vi "test SSL Client Valid Socket FD.vi"(8 "error in (no error)":errorcluster, 11 "TestCase in":refnum<class "test SSL Client.lvclass">) -> (0 "error out":errorcluster, 3 "TestCase out":refnum<class "test SSL Client.lvclass">)   [LabVIEW 2013, in "test SSL Client.lvclass"]
uses:
  test SSL Client.lvclass
  <vilib>/addons/_JKI Toolkits/VI Tester/TestCase.llb/TestCase.lvclass
  SSL_Lib/BIO/BIO.lvclass
  SSL_Lib/SSL-Context/SSL-Context.lvclass
  SSL_Lib/SSL/SSL.lvclass
  SSL_Lib/SSL/SSL_Mode.ctl
  suite SSL Client/suite SSL Client/SSL Context.vi
  suite SSL Client/suite SSL Client/suite SSL Client.lvclass
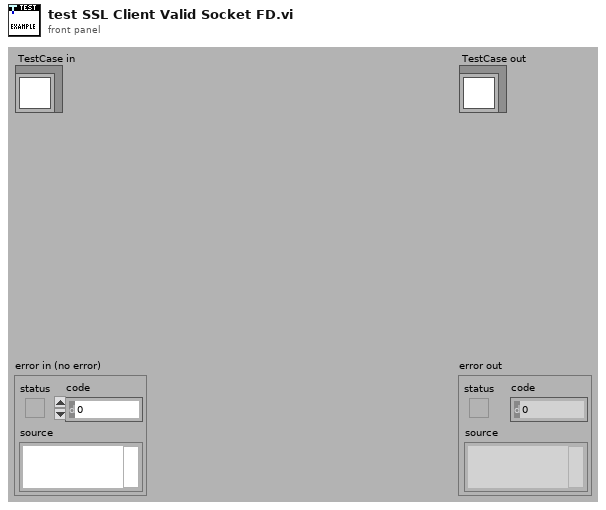
[diagram p1: front panel]
types:
  T1 = typedef "SSL_Lib.lvlib/SSL.lvclass/SSL_Mode.ctl" = i32
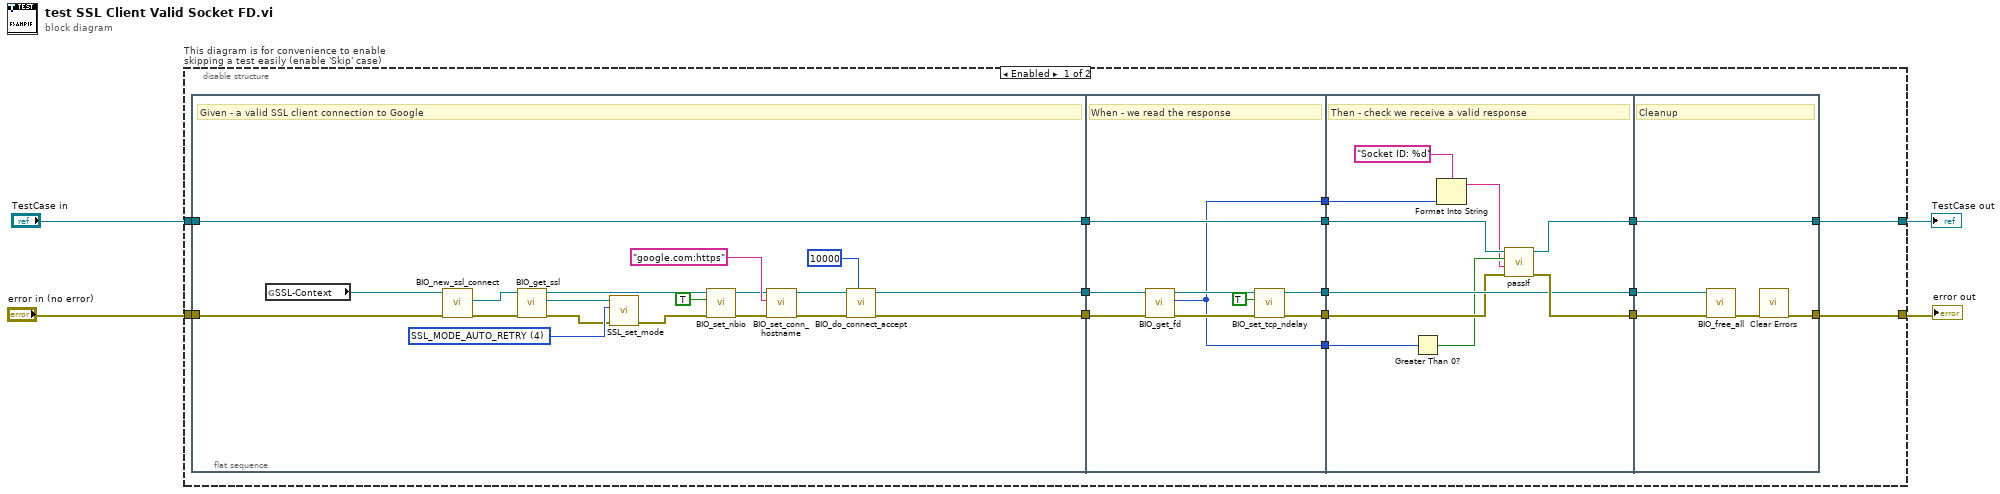
[diagram p0: block diagram]
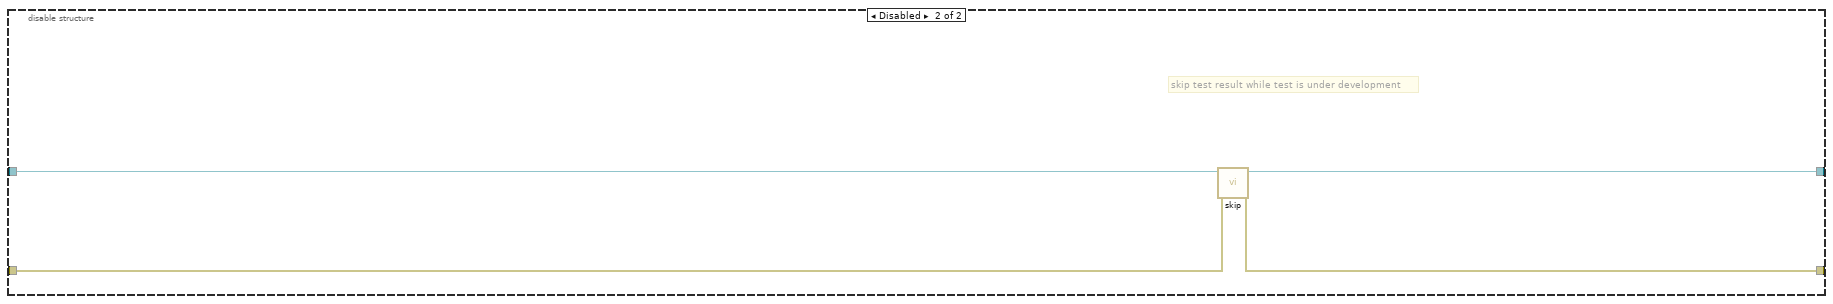
[diagram p2: hidden frame]
diagram:
  n1 = disable-structure "This diagram is for convenience to enable skipping a test easily (enable 'Skip' case)" shown="Enabled" {
    disable-tunnel: "TestCase in" -> [w14 w66]
    disable-tunnel: [w13 w64] -> w1
    disable-tunnel: [w12 w65] -> w3
    disable-tunnel: "error in (no error)" -> [w15 w63]
    frame Enabled {
      n2 = flat-sequence {
        tunnel: w15 -> [w28]
        tunnel: w14 -> [w35]
        tunnel: [w35] -> w19
        tunnel: [w21] -> w9
        tunnel: [w20] -> w8
        tunnel: [w47] -> w18
        tunnel: w19 -> [w47]
        tunnel: [w46] -> w11
        tunnel: w9 -> [w45]
        tunnel: w8 -> [w42]
        tunnel: [w41] -> w7
        tunnel: [w41] -> w6
        tunnel: [w39] -> w5
        tunnel: [w56] -> w17
        tunnel: [w55] -> w16
        tunnel: w18 -> [w57]
        tunnel: w11 -> [w54]
        tunnel: [w54] -> w10
        tunnel: w7 -> [w53]
        tunnel: w6 -> [w52]
        tunnel: w5 -> [w51]
        tunnel: [w58] -> w12
        tunnel: [w62] -> w13
        tunnel: w17 -> [w62]
        tunnel: w16 -> [w61]
        tunnel: w10 -> [w59]
        frame #0 {
          w30 = T1 4 items=["None"=0, "SSL_MODE_ENABLE_PARTIAL_WRITE"=1, "SSL_MODE_ACCEPT_MOVING_WRITE_BUFFER"=2, "SSL_MODE_AUTO_RETRY"=4, "SSL_MODE_RELEASE_BUFFERS"=16, "SSL_MODE_SEND_FALLBACK_SCSV"=128] ("Mode")
          # "Given - a valid SSL client connection to Google"
          n3 = global read "SSL Context.vi" "SSL-Context"() -> (w27:refnum<class "SSL-Context.lvclass">)
          n4 = call "BIO_new_ssl_connect.vi"("error in (no error)"=w28, "SSL-Context in"=w27) -> ("error out"=w32:errorcluster, "BIO out"=w33:refnum<class "BIO.lvclass">)  [unwired: 7 in, 1 out]
          n5 = call "BIO_get_ssl.vi"("error in (no error)"=w32, "BIO in"=w33) -> ("error out"=w29:errorcluster, "SSL out"=w31:refnum<class "SSL.lvclass">, "BIO out"=w22:refnum<class "BIO.lvclass">)  [unwired: 7 in]
          n6 = call "SSL_set_mode.vi"("error in (no error)"=w29, "Mode"=w30, "SSL in"=w31) -> ("error out"=w25:errorcluster)  [unwired: 7 in, 1 out]
          n7 = call "BIO_set_nbio.vi"("error in (no error)"=w25, "Non-Blocking?"=TRUE, "BIO in"=w22) -> ("error out"=w23:errorcluster, "BIO out"=w24:refnum<class "BIO.lvclass">)  [unwired: 7 in]
          n8 = call "BIO_set_conn_hostname.vi"("error in (no error)"=w23, "Hostname"="google.com:https", "BIO in"=w24) -> ("error out"=w37:errorcluster, "BIO out"=w34:refnum<class "BIO.lvclass">)  [unwired: 7 in]
          n9 = call "BIO_do_connect_accept.vi"("Timeout (10000ms)"=u32 10000, "error in (no error)"=w37, "BIO in"=w34) -> ("error out"=w21:errorcluster, "BIO out"=w20:refnum<class "BIO.lvclass">)  [unwired: 7 in]
        }
        frame #1 {
          # "When - we read the response"
          n10 = call "BIO_get_fd.vi"("error in (no error)"=w45, "BIO in"=w42) -> ("error out"=w44:errorcluster, "socket fd"=w41:i32, "BIO out"=w43:refnum<class "BIO.lvclass">)  [unwired: 7 in]
          n11 = call "BIO_set_tcp_ndelay.vi"("error in (no error)"=w44, "No Delay?"=TRUE, "BIO in"=w43) -> ("error out"=w39:errorcluster, "BIO out"=w46:refnum<class "BIO.lvclass">)  [unwired: 7 in]
        }
        frame #2 {
          # "Then - check we receive a valid response"
          n12 = Greater Than 0?(x=w52) -> (x > 0?=w50:bool)
          n13 = Format Into String(format string="Socket ID: %d", w53) -> (resulting string=w48:string)  [unwired: 2 in, 1 out]
          n14 = call-dynamic "passIf.vi"("error in (no error)"=w51, "message (\"\")"=w48, "pass"=w50, "TestCase in"=w57) -> ("error out"=w55:errorcluster, "TestCase out"=w56:refnum<class "test SSL Client.lvclass">)  [unwired: 6 in]
        }
        frame #3 {
          # "Cleanup"
          n15 = call "BIO_free_all.vi"("error in (no error)"=w61, "BIO in"=w59) -> ("error out"=w60:errorcluster)  [unwired: 9 in]
          n16 = call <vilib>:"Clear Errors.vi"("error in (no error)"=w60) -> ("error out"=w58:errorcluster)  [unwired: 5 in, 1 out]
        }
      }
    }
    frame Disabled {
      # "skip test result while test is under development"
      n17 = call <vilib>:"skip.vi"("error in (no error)"=w63, "TestCase in"=w66) -> ("error out"=w65:errorcluster, "TestCase out"=w64:refnum<class "test SSL Client.lvclass">)  [unwired: 8 in]
    }
  }
  "error out" <- w3
  "TestCase out" <- w1
